vi "Create_waveform.vi"(9 "time":timestamp, 10 "Step Pos":dbl, 11 "ADC Pos":dbl) -> (3 "waveform_array":waveform(dbl)[](array[waveform])=[{"t0"=timestamp(0 s since 1904-01-01), "dt"=1.0, "Y"=[]}, {"t0"=timestamp(3732035173.078092 s since 1904-01-01), "dt"=1.0, "Y"=[302.8589782714844], "attributes"=variant("NI_ChannelName"=variant(string "T1"))}])   [LabVIEW 2019]
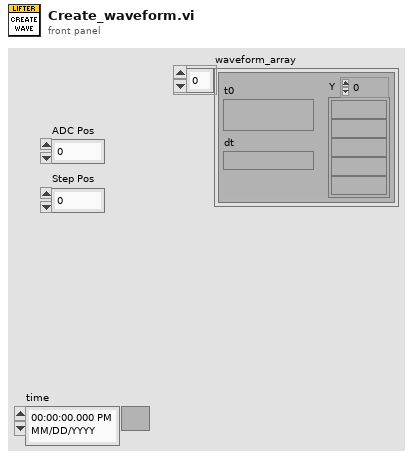
[diagram p1: front panel]
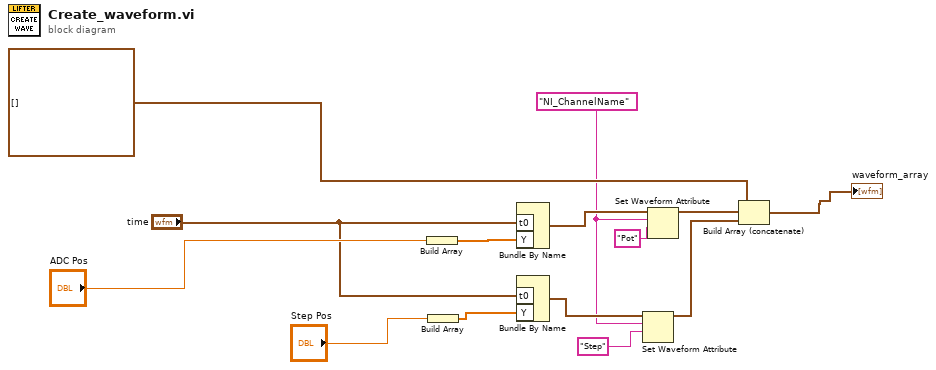
[diagram p0: block diagram]
diagram:
  w2 = "NI_ChannelName" ("name")
  n1 = Build Array("ADC Pos") -> (w12:dbl[])
  n2 = Build Array("Step Pos") -> (w8:dbl[])
  n3 = Bundle By Name("t0"="time", "Y"=w12) -> (w3:waveform(dbl))  [unwired: 1 in]
  n4 = Bundle By Name("t0"="time", "Y"=w8) -> (w6:waveform(dbl))  [unwired: 1 in]
  n5 = Set Waveform Attribute(5:"Step" ("name"), 6:w2, 7:w6) -> (3:w7:waveform(dbl))  [unwired: 1 in, 2 out]
  n6 = Set Waveform Attribute(5:"Pot" ("name"), 6:w2, 7:w3) -> (3:w4:waveform(dbl))  [unwired: 1 in, 2 out]
  n7 = Build Array (concatenate)(waveform(dbl)[] [], w4, w7) -> (→"waveform_array":waveform(dbl)[])
